vi "Get Idle.vi"(8 "error in (no error)":errorcluster, 11 "Scorer in":refnum<class "Scorer.lvclass">) -> (0 "error out":errorcluster, 2 "Idle":bool, 3 "Scorer out":refnum<class "Scorer.lvclass">)   [LabVIEW 2020, in "Summer of LabVIEW.lvlib" / "Scorer.lvclass"]
uses:
  Scorer.lvclass
  Scorer.lvclass/Scorer.ctl
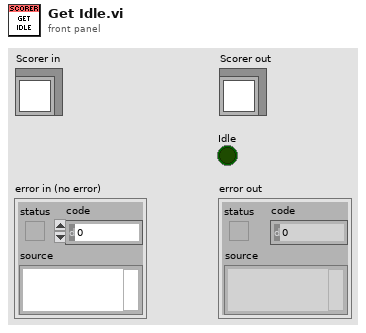
[diagram p1: front panel]
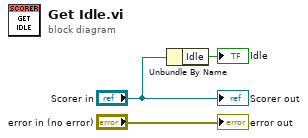
[diagram p0: block diagram]
diagram:
  n1 = Unbundle By Name("Scorer in") -> ("Idle"=→"Idle":bool)
  "error out" <- "error in (no error)"
  "Scorer out" <- "Scorer in"
